vi "ABR-Estimate Threshold.vi"(0 "Analysis in":T1) -> (4 "Analysis out":T1)   [LabVIEW 2020]
uses:
  epl-vi-lib/Utility VIs/Math VIs/interp1.vi
  Typedefs/ABR-Analysis State.ctl
  Threshold Estimation VIs/ABR3-Threshold Estimation Result.ctl
panel:
  in  "CorrCoef Criterion":dbl=0.5
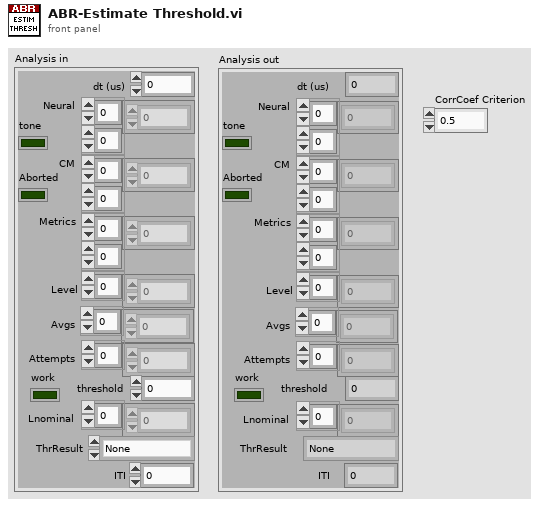
[diagram p1: front panel]
types:
  T1 = typedef "ABR-Analysis State.ctl" = cluster{"dt (us)":dbl, "Neural":dbl[][], "CM":dbl[][], "Metrics":dbl[][], "Level":dbl[], "Avgs":i32[], "Attempts":i32[], "Aborted":bool, "threshold":dbl, "Lnominal":dbl[], "tone":bool, "work":bool, "ThrResult":T2, "ITI":dbl}
  T2 = typedef "ABR3-Threshold Estimation Result.ctl" = enum16{"None", "Power", "Sigmoid", "Power (noisy)", "Suprathreshold", "Invalid"}
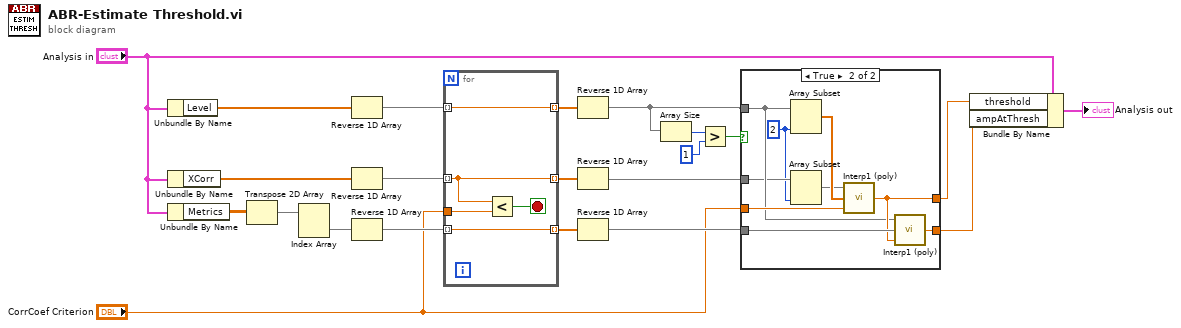
[diagram p0: block diagram]
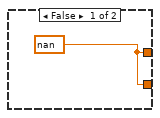
[diagram p2: hidden frame]
diagram:
  n1 = Unbundle By Name("Analysis in") -> ("Level"=w21:dbl[])
  n2 = Unbundle By Name("Analysis in") -> ("XCorr"=w22:dbl[])
  n3 = Unbundle By Name("Analysis in") -> ("Metrics"=w18:dbl[][])
  n4 = Transpose 2D Array(2D array=w18) -> (transposed array=w17:dbl[][])
  n5 = Index Array(array=w17) -> (element=w16:dbl[])  [unwired: 2 in]
  n6 = Reverse 1D Array(array=w21) -> (reversed array=w15:dbl[])
  n7 = Reverse 1D Array(array=w22) -> (reversed array=w14:dbl[])
  n8 = Reverse 1D Array(array=w16) -> (reversed array=w13:dbl[])
  n9 = for {
    tunnel: w14 -> [w26] mode=indexing
    tunnel: [w27] -> w12 mode=indexing
    tunnel: w15 -> [w27] mode=indexing
    tunnel: [w26] -> w11 mode=indexing
    tunnel: "CorrCoef Criterion" -> [w25]
    tunnel: w13 -> [w24] mode=indexing
    tunnel: [w24] -> w10 mode=indexing
    stop <- w23 stop-if-true
    n10 = Less?(x=w26, y=w25) -> (x < y?=w23:bool)
  }
  n11 = Reverse 1D Array(array=w12) -> (reversed array=w7:dbl[])
  n12 = Reverse 1D Array(array=w11) -> (reversed array=w6:dbl[])
  n13 = Reverse 1D Array(array=w10) -> (reversed array=w5:dbl[])
  n14 = Array Size(array=w7) -> (size(s)=w9:i32)
  n15 = Greater?(x=w9, y=1) -> (0:w1:bool)
  n16 = case shown="True" w1 {
    tunnel: [w28 w35] -> w3
    tunnel: w7 -> [_ w33]
    tunnel: w6 -> [_ w32]
    tunnel: "CorrCoef Criterion" -> [_ w37]
    tunnel: w5 -> [_ w36]
    tunnel: [w28 w34] -> w2
    frame False {
      w28 = nan
    }
    frame True {
      w31 = 2
      n17 = Array Subset(array=w33, length=w31) -> (w30:dbl[])  [unwired: 1 in]
      n18 = Array Subset(array=w32, length=w31) -> (w29:dbl[])  [unwired: 1 in]
      n19 = call-poly "Interp1 (poly).vi"("U"=w37, "Y"=w30, "X"=w29) -> ("V"=w35:dbl)
      n20 = call-poly "Interp1 (poly).vi"("U"=w35, "Y"=w36, "X"=w33) -> ("V"=w34:dbl)
    }
  }
  n21 = Bundle By Name(cluster="Analysis in", "threshold"=w3, "ampAtThresh"=w2) -> (→"Analysis out":T1)
